vi "Container State.vi"(8 "error in (no error)":errorcluster, 11 "Container in":refnum<class "Container.lvclass">) -> (0 "error out":errorcluster, 3 "Container out":refnum<class "Container.lvclass">)   [LabVIEW 2016]
uses:
  Controls/Shutter States.ctl
  Shutter.lvclass
  Controls/Operational Modes.ctl
  Container.lvclass
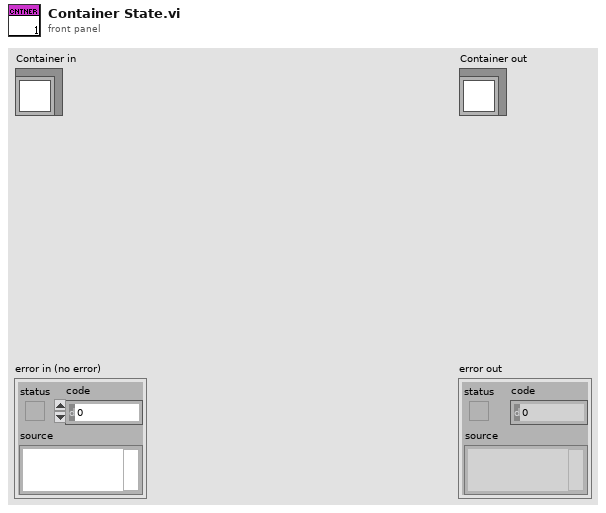
[diagram p1: front panel]
types:
  T1 = typedef "Operational Modes.ctl" = enum16{"Sci", "Sci-LFC", "Solar", "Solar-LFC", "LFC", "LFC-Sim", "LFC-Both", "ThAr", "ThAr-LFC", "Flat", "ExtFlat", "ExtFlat-Sim", "ExtFlat-Both", "Qtz", "ExtQtz", "ExtQtz-Sim", "ExtQtz-Both", "Dark", "Manual", "Off"}
  T2 = typedef "Shutter States.ctl" = enum16{"Open", "Close", "Wait", "Off", "Arm", "Idle"}
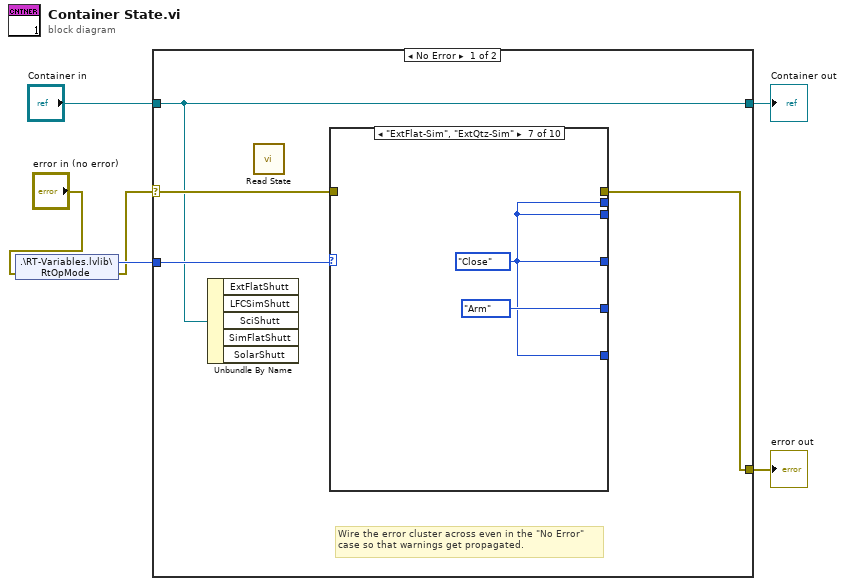
[diagram p0: block diagram]
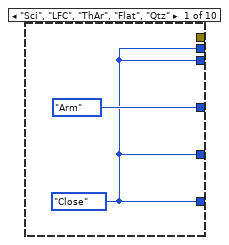
[diagram p2: hidden frame]
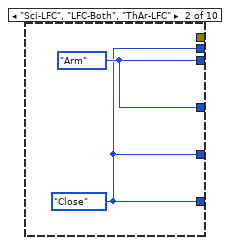
[diagram p3: hidden frame]
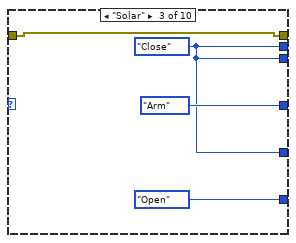
[diagram p4: hidden frame]
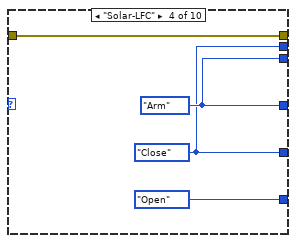
[diagram p5: hidden frame]
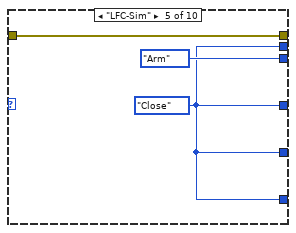
[diagram p6: hidden frame]
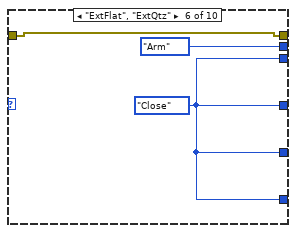
[diagram p7: hidden frame]
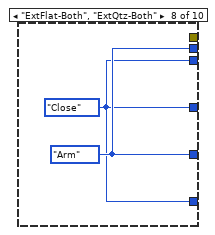
[diagram p8: hidden frame]
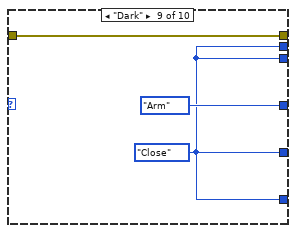
[diagram p9: hidden frame]
diagram:
  n1 = shared-variable ".\\RT-Variables.lvlib\\RtOpMode"(error in="error in (no error)") -> (w3:T1, error out=w1:errorcluster)
  n2 = case shown="No Error" w1 {
    selector: w1 -> [w10 w38]
    tunnel: [w9 w38] -> w6
    tunnel: [w7 w37] -> w4
    tunnel: "Container in" -> [w7 w37]
    tunnel: w3 -> [w8 _]
    frame No Error {
      # "Wire the error cluster across even in the \"No Error\"\ncase so that warnings get propagated."
      n3 = Unbundle By Name(w7) -> ()  [unwired: 5 out]
      n4 = call-dynamic "Read State.vi"() -> ()  [unwired: 9 in, 3 out]
      n5 = case shown="\"ExtFlat-Sim\", \"ExtQtz-Sim\"" w8 {
        tunnel: [Shutter_States."Arm" ("Set") w14 Shutter_States."Arm" ("Set") w22 w24 w27 w29 w31 Shutter_States."Arm" ("Set") _] -> _
        tunnel: [w11 w14 w17 w22 Shutter_States."Arm" ("Set") w27 w29 w31 w34 _] -> _
        tunnel: [w11 w13 w17 w21 w24 Shutter_States."Arm" ("Set") w29 w32 w34 _] -> _
        tunnel: [w11 w13 w17 w21 w24 w27 Shutter_States."Arm" ("Set") w32 w34 _] -> _
        tunnel: [w11 w13 Shutter_States."Open" ("Set") Shutter_States."Open" ("Set") w24 w27 w29 w31 w34 _] -> _
        tunnel: w10 -> [_ _ w15 w19 w23 w26 _ _ w33 w36]
        tunnel: [_ _ w15 w19 w23 w26 _ _ w33 w36] -> w9
        frame "Sci", "LFC", "ThAr", "Flat", "Qtz" {
          w11 = Shutter_States."Close" ("Set")
        }
        frame "Sci-LFC", "LFC-Both", "ThAr-LFC" {
          w13 = Shutter_States."Close" ("Set")
          w14 = Shutter_States."Arm" ("Set")
        }
        frame "Solar" {
          w17 = Shutter_States."Close" ("Set")
        }
        frame "Solar-LFC" {
          w21 = Shutter_States."Close" ("Set")
          w22 = Shutter_States."Arm" ("Set")
        }
        frame "LFC-Sim" {
          w24 = Shutter_States."Close" ("Set")
        }
        frame "ExtFlat", "ExtQtz" {
          w27 = Shutter_States."Close" ("Set")
        }
        frame "ExtFlat-Sim", "ExtQtz-Sim" {
          w29 = Shutter_States."Close" ("Set")
        }
        frame "ExtFlat-Both", "ExtQtz-Both" {
          w31 = Shutter_States."Close" ("Set")
          w32 = Shutter_States."Arm" ("Set")
        }
        frame "Dark" {
          w34 = Shutter_States."Close" ("Set")
        }
        frame "Off", Default {
        }
      }
    }
    frame Error {
    }
  }
  "error out" <- w6
  "Container out" <- w4
